vi "AIKoeffSortieren.vi"(3 "Modul3/AI koeff":dbl[][](array[numeric]), 4 "Modul2/AI koeff":dbl[][](array[numeric]), 5 "Modul1/AI koeff":dbl[][](array[numeric])) -> (0 "P0":dbl[](array[numeric]), 1 "P1":dbl[](array[numeric]), 2 "P2":dbl[](array[numeric]))   [LabVIEW 2017]
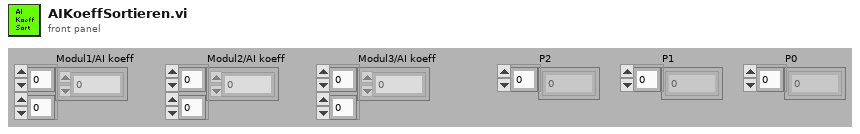
[diagram p1: front panel]
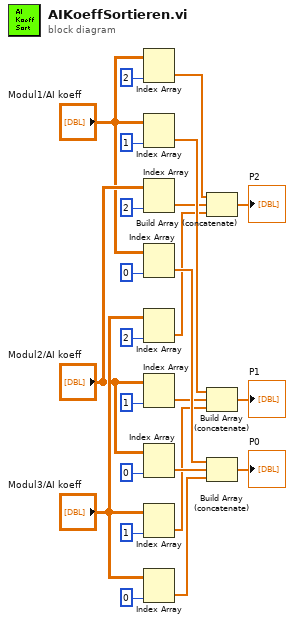
[diagram p0: block diagram]
diagram:
  n1 = Index Array(array="Modul1/AI koeff", index (col)=2 ("Deaktivierter Index (Spalte)")) -> (element=w13:dbl[])  [unwired: 1 in]
  n2 = Index Array(array="Modul1/AI koeff", index (col)=1 ("Deaktivierter Index (Spalte)")) -> (element=w16:dbl[])  [unwired: 1 in]
  n3 = Index Array(array="Modul2/AI koeff", index (col)=2 ("Deaktivierter Index (Spalte)")) -> (element=w14:dbl[])  [unwired: 1 in]
  n4 = Index Array(array="Modul1/AI koeff", index (col)=0 ("Deaktivierter Index (Spalte)")) -> (element=w19:dbl[])  [unwired: 1 in]
  n5 = Index Array(array="Modul3/AI koeff", index (col)=2 ("Deaktivierter Index (Spalte)")) -> (element=w15:dbl[])  [unwired: 1 in]
  n6 = Index Array(array="Modul2/AI koeff", index (col)=1 ("Deaktivierter Index (Spalte)")) -> (element=w17:dbl[])  [unwired: 1 in]
  n7 = Index Array(array="Modul2/AI koeff", index (col)=0 ("Deaktivierter Index (Spalte)")) -> (element=w20:dbl[])  [unwired: 1 in]
  n8 = Index Array(array="Modul3/AI koeff", index (col)=1 ("Deaktivierter Index (Spalte)")) -> (element=w18:dbl[])  [unwired: 1 in]
  n9 = Index Array(array="Modul3/AI koeff", index (col)=0 ("Deaktivierter Index (Spalte)")) -> (element=w21:dbl[])  [unwired: 1 in]
  n10 = Build Array (concatenate)(w13, w14, w15) -> (→"P2":dbl[])
  n11 = Build Array (concatenate)(w16, w17, w18) -> (→"P1":dbl[])
  n12 = Build Array (concatenate)(w19, w20, w21) -> (→"P0":dbl[])
